vi "3.Rtde.vi"() -> ()   [LabVIEW 2016]
uses:
  UnderAutomation.UniversalRobots/UnderAutomation.UniversalRobots.lvlib
panel:
  in  "Slide":dbl(slide) min=0.0 max=1.0 step=0.01 scale=0.0..1.0
  in  "stop":bool
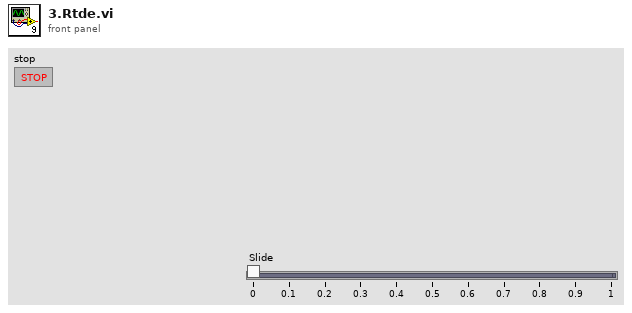
[diagram p1: front panel]
types:
  T1 = cluster{"ConfigurableDigitalOutput":u8, "ConfigurableDigitalOutputMask":u8, "ExternalForceTorque":cluster{"X":dbl, "Y":dbl, "Z":dbl, "Rx":dbl, "Ry":dbl, "Rz":dbl}, "InputBitRegisters":cluster{"X64":bool, "X65":bool, "X66":bool, "X67":bool, "X68":bool, "X69":bool, "X70":bool, "X71":bool, "X72":bool, "X73":bool, "X74":bool, "X75":bool, "X76":bool, "X77":bool, "X78":bool, "X79":bool, "X80":bool, "X81":bool, "X82":bool, "X83":bool, "X84":bool, "X85":bool, "X86":bool, "X87":bool, "X88":bool, "X89":bool, "X90":bool, "X91":bool, "X92":bool, "X93":bool, "X94":bool, "X95":bool, "X96":bool, "X97":bool, "X98":bool, "X99":bool, "X100":bool, "X101":bool, "X102":bool, "X103":bool, "X104":bool, "X105":bool, "X106":bool, "X107":bool, "X108":bool, "X109":bool, "X110":bool, "X111":bool, "X112":bool, "X113":bool, "X114":bool, "X115":bool, "X116":bool, "X117":bool, "X118":bool, "X119":bool, "X120":bool, "X121":bool, "X122":bool, "X123":bool, "X124":bool, "X125":bool, "X126":bool, "X127":bool}, "InputBtRegisters0To31":u32, "InputBtRegisters32To63":u32, "InputDoubleRegisters":cluster{"X0":dbl, "X1":dbl, "X2":dbl, "X3":dbl, "X4":dbl, "X5":dbl, "X6":dbl, "X7":dbl, "X8":dbl, "X9":dbl, "X10":dbl, "X11":dbl, "X12":dbl, "X13":dbl, "X14":dbl, "X15":dbl, "X16":dbl, "X17":dbl, "X18":dbl, "X19":dbl, "X20":dbl, "X21":dbl, "X22":dbl, "X23":dbl, "X24":dbl, "X25":dbl, "X26":dbl, "X27":dbl, "X28":dbl, "X29":dbl, "X30":dbl, "X31":dbl, "X32":dbl, "X33":dbl, "X34":dbl, "X35":dbl, "X36":dbl, "X37":dbl, "X38":dbl, "X39":dbl, "X40":dbl, "X41":dbl, "X42":dbl, "X43":dbl, "X44":dbl, "X45":dbl, "X46":dbl, "X47":dbl}, "InputIntRegisters":cluster{"X0":i32, "X1":i32, "X2":i32, "X3":i32, "X4":i32, "X5":i32, "X6":i32, "X7":i32, "X8":i32, "X9":i32, "X10":i32, "X11":i32, "X12":i32, "X13":i32, "X14":i32, "X15":i32, "X16":i32, "X17":i32, "X18":i32, "X19":i32, "X20":i32, "X21":i32, "X22":i32, "X23":i32, "X24":i32, "X25":i32, "X26":i32, "X27":i32, "X28":i32, "X29":i32, "X30":i32, "X31":i32, "X32":i32, "X33":i32, "X34":i32, "X35":i32, "X36":i32, "X37":i32, "X38":i32, "X39":i32, "X40":i32, "X41":i32, "X42":i32, "X43":i32, "X44":i32, "X45":i32, "X46":i32, "X47":i32}, "SpeedSliderFraction":dbl, "SpeedSliderMask":u32, "StandardAnalogOutput0":dbl, "StandardAnalogOutput1":dbl, "StandardAnalogOutputMask":u8, "StandardAnalogOutputType":u8, "StandardDigitalOutput":u8, "StandardDigitalOutputMask":u8}
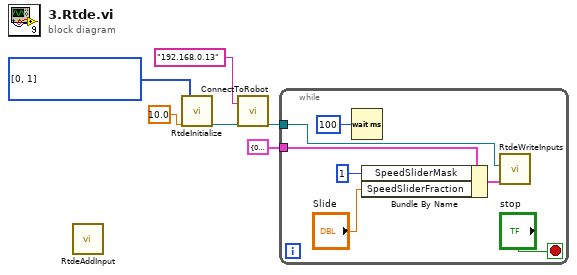
[diagram p0: block diagram]
diagram:
  w3 = i32[] [0, 1] items=["SpeedSliderMask", "SpeedSliderFraction", "StandardDigitalOutputMask", "ConfigurableDigitalOutputMask", "StandardDigitalOutput", "ConfigurableDigitalOutput", "StandardAnalogOutputMask", "StandardAnalogOutputType", "StandardAnalogOutput0", "StandardAnalogOutput1", "InputBtRegisters0To31", "InputBtRegisters32To63", "InputBitRegisters", "InputIntRegisters", "InputDoubleRegisters", "ExternalForceTorque"] ("InputData")
  n1 = call "RtdeAddInput.vi"() -> ()  [unwired: 10 in, 2 out]
  n2 = call "RtdeInitialize.vi"("Frequency"=10.0, "InputData"=w3) -> ("RTDE Connect Parameters"=w1:refnum<k24>)  [unwired: 16 in, 1 out]
  n3 = call "ConnectToRobot.vi"("ip"="192.168.0.13", "RTDE Connect Parameters"=w1) -> ("Rtde"=w5:refnum<k24>)  [unwired: 12 in, 5 out]
  n4 = while {
    tunnel: w5 -> [w13]
    tunnel: T1 {"ConfigurableDigitalOutput"=0, "ConfigurableDigitalOutputMask"=0, "ExternalForceTorque"={"X"=0.0, "Y"=0.0, "Z"=0.0, "Rx"=0.0, "Ry"=0.0, "Rz"=0.0}, "InputBitRegisters"={"X64"=FALSE, "X65"=FALSE, "X66"=FALSE, "X67"=FALSE, "X68"=FALSE, "X69"=FALSE, "X70"=FALSE, "X71"=FALSE, "X72"=FALSE, "X73"=FALSE, "X74"=FALSE, "X75"=FALSE, "X76"=FALSE, "X77"=FALSE, "X78"=FALSE, "X79"=FALSE, "X80"=FALSE, "X81"=FALSE, "X82"=FALSE, "X83"=FALSE, "X84"=FALSE, "X85"=FALSE, "X86"=FALSE, "X87"=FALSE, "X88"=FALSE, "X89"=FALSE, "X90"=FALSE, "X91"=FALSE, "X92"=FALSE, "X93"=FALSE, "X94"=FALSE, "X95"=FALSE, "X96"=FALSE, "X97"=FALSE, "X98"=FALSE, "X99"=FALSE, "X100"=FALSE, "X101"=FALSE, "X102"=FALSE, "X103"=FALSE, "X104"=FALSE, "X105"=FALSE, "X106"=FALSE, "X107"=FALSE, "X108"=FALSE, "X109"=FALSE, "X110"=FALSE, "X111"=FALSE, "X112"=FALSE, "X113"=FALSE, "X114"=FALSE, "X115"=FALSE, "X116"=FALSE, "X117"=FALSE, "X118"=FALSE, "X119"=FALSE, "X120"=FALSE, "X121"=FALSE, "X122"=FALSE, "X123"=FALSE, "X124"=FALSE, "X125"=FALSE, "X126"=FALSE, "X127"=FALSE}, "InputBtRegisters0To31"=0, "InputBtRegisters32To63"=0, "InputDoubleRegisters"={"X0"=0.0, "X1"=0.0, "X2"=0.0, "X3"=0.0, "X4"=0.0, "X5"=0.0, "X6"=0.0, "X7"=0.0, "X8"=0.0, "X9"=0.0, "X10"=0.0, "X11"=0.0, "X12"=0.0, "X13"=0.0, "X14"=0.0, "X15"=0.0, "X16"=0.0, "X17"=0.0, "X18"=0.0, "X19"=0.0, "X20"=0.0, "X21"=0.0, "X22"=0.0, "X23"=0.0, "X24"=0.0, "X25"=0.0, "X26"=0.0, "X27"=0.0, "X28"=0.0, "X29"=0.0, "X30"=0.0, "X31"=0.0, "X32"=0.0, "X33"=0.0, "X34"=0.0, "X35"=0.0, "X36"=0.0, "X37"=0.0, "X38"=0.0, "X39"=0.0, "X40"=0.0, "X41"=0.0, "X42"=0.0, "X43"=0.0, "X44"=0.0, "X45"=0.0, "X46"=0.0, "X47"=0.0}, "InputIntRegisters"={"X0"=0, "X1"=0, "X2"=0, "X3"=0, "X4"=0, "X5"=0, "X6"=0, "X7"=0, "X8"=0, "X9"=0, "X10"=0, "X11"=0, "X12"=0, "X13"=0, "X14"=0, "X15"=0, "X16"=0, "X17"=0, "X18"=0, "X19"=0, "X20"=0, "X21"=0, "X22"=0, "X23"=0, "X24"=0, "X25"=0, "X26"=0, "X27"=0, "X28"=0, "X29"=0, "X30"=0, "X31"=0, "X32"=0, "X33"=0, "X34"=0, "X35"=0, "X36"=0, "X37"=0, "X38"=0, "X39"=0, "X40"=0, "X41"=0, "X42"=0, "X43"=0, "X44"=0, "X45"=0, "X46"=0, "X47"=0}, "SpeedSliderFraction"=0.0, "SpeedSliderMask"=0, "StandardAnalogOutput0"=0.0, "StandardAnalogOutput1"=0.0, "StandardAnalogOutputMask"=0, "StandardAnalogOutputType"=0, "StandardDigitalOutput"=0, "StandardDigitalOutputMask"=0} ("Data") -> [w12]
    stop <- "stop" stop-if-true
    n5 = Wait (ms)(milliseconds to wait=u32 100) -> ()  [unwired: 1 out]
    n6 = Bundle By Name(cluster=w12, "SpeedSliderMask"=u32 1, "SpeedSliderFraction"="Slide") -> (w11:T1)
    n7 = call "RtdeWriteInputs.vi"("Data"=w11, "Rtde"=w13) -> ()  [unwired: 9 in, 1 out]
  }
